vi "Saved Checker.vi"(1 "comp A":T4={"Trajectory Data"=[], "Updated Waypoints"=[], {"Sample Period (s)"=0.0, "Limits"={"Velocity (fps)"=6.0, "Accel (fps^2)"=15.0, "Jerk (fps^3)"=150.0, "StoopidFast (fps)"=6.0}, "Conditions"={"vInitial (fps)"=0.0, "vFinal (fps)"=0.0}, "Angular Accelerations"={"Angular \nAccelerations"=[], "Override Limits?"=[]}}, "Commands"=[]} {"?"."Limits"."StoopidFast (fps)" min=0.0; "?"."Limits"."Jerk (fps^3)" min=0.0 step=1.0; "?"."Limits"."Accel (fps^2)" min=0.0; "?"."Limits"."Velocity (fps)" min=0.0}, 2 "comp B":T5={"Trajectory Data"=[], "Points"=[], {"Sample Period (s)"=0.0, "Limits"={"Velocity (fps)"=6.0, "Accel (fps^2)"=15.0, "Jerk (fps^3)"=150.0, "StoopidFast (fps)"=6.0}, "Conditions"={"vInitial (fps)"=0.0, "vFinal (fps)"=0.0}, "Angular Accelerations"={"Angular \nAccelerations"=[], "Override Limits?"=[]}}, "Commands"=[]} {"?"."Limits"."StoopidFast (fps)" min=0.0; "?"."Limits"."Jerk (fps^3)" min=0.0 step=1.0; "?"."Limits"."Accel (fps^2)" min=0.0; "?"."Limits"."Velocity (fps)" min=0.0}) -> (0 "Unsaved":bool)   [LabVIEW 2019]
uses:
  Limits.ctl
  Command Stuff/Single Cmd Info.ctl
  <vilib>/picture/picture.llb/imagedata.ctl
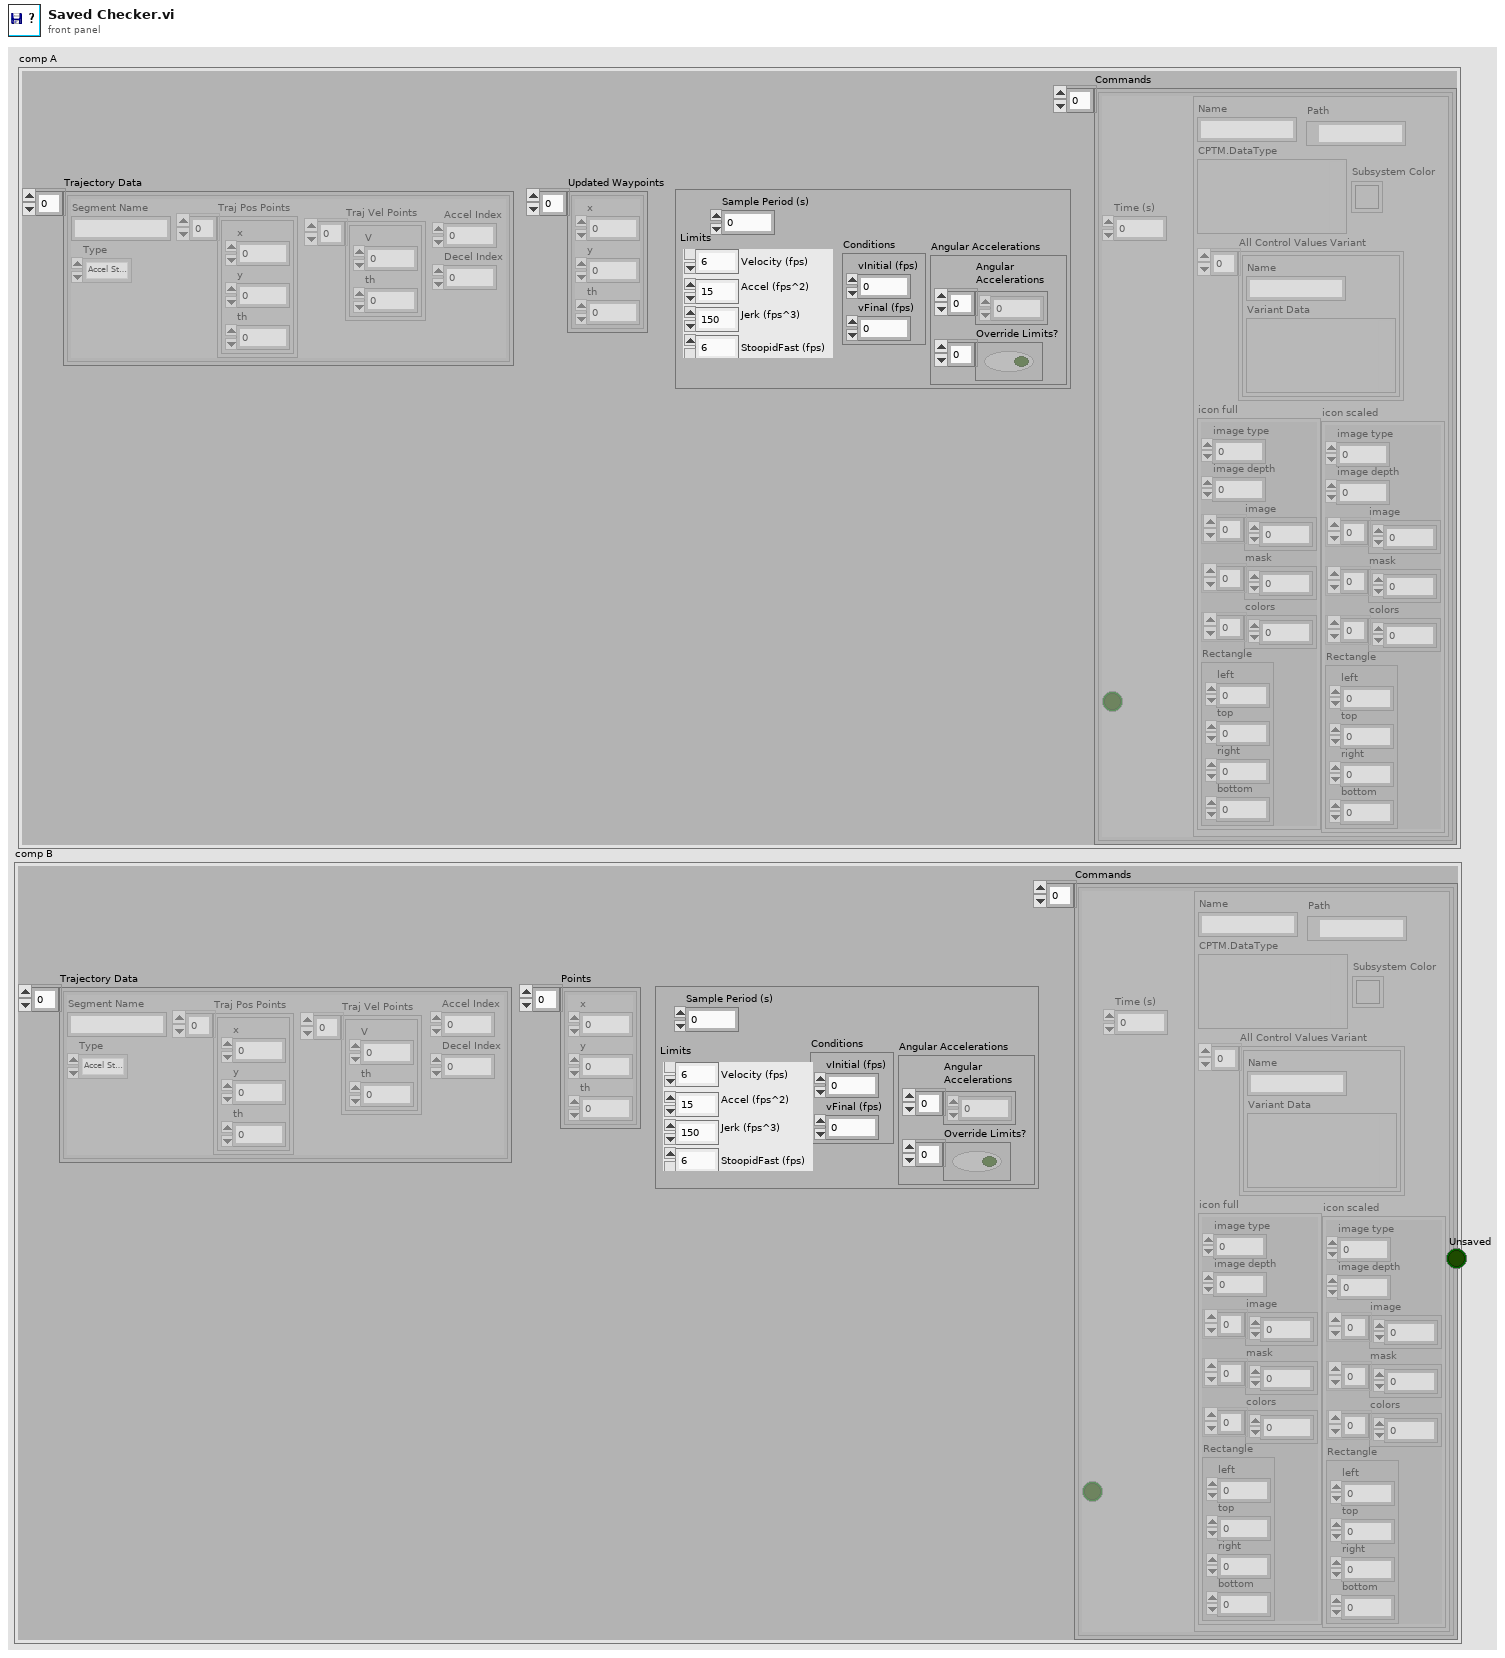
[diagram p1: front panel]
types:
  T1 = typedef "Limits.ctl" = cluster{"Velocity (fps)":dbl, "Accel (fps^2)":dbl, "Jerk (fps^3)":dbl, "StoopidFast (fps)":dbl}
  T2 = typedef "Single Cmd Info.ctl" = cluster{"Name":string, "CPTM.DataType":variant, "All Control Values Variant":cluster{"Name":string, "Variant Data":variant}[], "icon full":T3, "icon scaled":T3, "Path":path, "Subsystem Color":u32}
  T3 = typedef "imagedata.ctl" = cluster{"image type":i32, "image depth":i32, "image":u8[], "mask":u8[], "colors":u32[], "Rectangle":cluster{"left":i16, "top":i16, "right":i16, "bottom":i16}}
  T4 = cluster{"Trajectory Data":cluster{"Segment Name":string, "Type":enum16{"Accel Straight", "Const Straight", "Blend", "Circle"}, "Traj Pos Points":cluster{"x":dbl, "y":dbl, "th":dbl}[], "Traj Vel Points":cluster{"V":dbl, "th":dbl}[], "Accel Index":i32, "Decel Index":i32}[], "Updated Waypoints":cluster{"x":dbl, "y":dbl, "th":dbl}[], cluster{"Sample Period (s)":dbl, "Limits":T1, "Conditions":cluster{"vInitial (fps)":dbl, "vFinal (fps)":dbl}, "Angular Accelerations":cluster{"Angular \nAccelerations":dbl[], "Override Limits?":bool[]}}, "Commands":cluster{"Time (s)":dbl, T2, bool}[]}
  T5 = cluster{"Trajectory Data":cluster{"Segment Name":string, "Type":enum16{"Accel Straight", "Const Straight", "Blend", "Circle"}, "Traj Pos Points":cluster{"x":dbl, "y":dbl, "th":dbl}[], "Traj Vel Points":cluster{"V":dbl, "th":dbl}[], "Accel Index":i32, "Decel Index":i32}[], "Points":cluster{"x":dbl, "y":dbl, "th":dbl}[], cluster{"Sample Period (s)":dbl, "Limits":T1, "Conditions":cluster{"vInitial (fps)":dbl, "vFinal (fps)":dbl}, "Angular Accelerations":cluster{"Angular \nAccelerations":dbl[], "Override Limits?":bool[]}}, "Commands":cluster{"Time (s)":dbl, T2, bool}[]}
  T6 = cluster{"Segment Name":string, "Type":enum16{"Accel Straight", "Const Straight", "Blend", "Circle"}, "Traj Pos Points":cluster{"x":dbl, "y":dbl, "th":dbl}[], "Traj Vel Points":cluster{"V":dbl, "th":dbl}[], "Accel Index":i32, "Decel Index":i32}[]
  T7 = cluster{"Sample Period (s)":dbl, "Limits":T1, "Conditions":cluster{"vInitial (fps)":dbl, "vFinal (fps)":dbl}, "Angular Accelerations":cluster{"Angular \nAccelerations":dbl[], "Override Limits?":bool[]}}
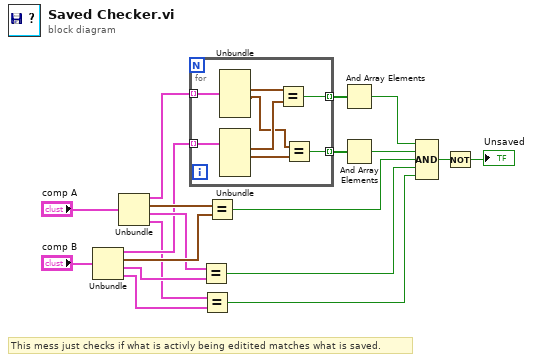
[diagram p0: block diagram]
diagram:
  # "This mess just checks if what is activly being editited matches what is saved."
  n1 = Unbundle("comp B") -> ("Trajectory Data"=w12:T6, "Points"=w16:cluster{"x":dbl, "y":dbl, "th":dbl}[], w13:T7, "Commands"=w3:cluster{"Time (s)":dbl, T2, bool}[])
  n2 = Unbundle("comp A") -> ("Trajectory Data"=w14:T6, "Updated Waypoints"=w17:cluster{"x":dbl, "y":dbl, "th":dbl}[], w15:T7, "Commands"=w2:cluster{"Time (s)":dbl, T2, bool}[])
  n3 = for {
    tunnel: w14 -> [w27] mode=indexing
    tunnel: w12 -> [w26] mode=indexing
    tunnel: [w21] -> w11 mode=indexing
    tunnel: [w20] -> w10 mode=indexing
    n4 = Unbundle(w27) -> ("Traj Pos Points"=w25:cluster{"x":dbl, "y":dbl, "th":dbl}[], "Traj Vel Points"=w22:cluster{"V":dbl, "th":dbl}[])  [unwired: 4 out]
    n5 = Unbundle(w26) -> ("Traj Pos Points"=w24:cluster{"x":dbl, "y":dbl, "th":dbl}[], "Traj Vel Points"=w23:cluster{"V":dbl, "th":dbl}[])  [unwired: 4 out]
    n6 = Equal?(x=w25, y=w24) -> (x = y?=w21:bool)
    n7 = Equal?(x=w22, y=w23) -> (x = y?=w20:bool)
  }
  n8 = Equal?(x=w15, y=w13) -> (x = y?=w6:bool)
  n9 = Equal?(x=w2, y=w3) -> (x = y?=w1:bool)
  n10 = Equal?(x=w17, y=w16) -> (x = y?=w7:bool)
  n11 = And Array Elements(Boolean array=w11) -> (logical AND=w9:bool)
  n12 = And Array Elements(Boolean array=w10) -> (logical AND=w8:bool)
  n13 = Compound Arithmetic op=AND(w9, w8, w7, w6, w1) -> (w5:bool)
  n14 = Not(x=w5) -> (.not. x?=→"Unsaved":bool)
